vi "CRYSet Cursor in Default Position.vi"(8 "Intensity Graph Ref":refnum<vi>, 9 "Wave Graph Ref":refnum<vi>, 10 "XY Graph Ref":refnum<vi>, 11 "Graph Type":string) -> ()   [LabVIEW 2013]
uses:
  <vilib>/Utility/miscctls.llb/LVPointDoubleTypeDef.ctl
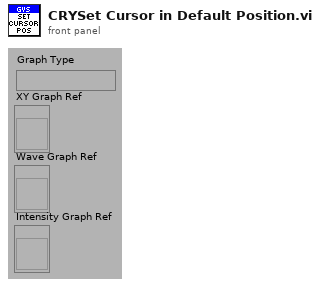
[diagram p1: front panel]
types:
  T1 = typedef "LVPointDoubleTypeDef.ctl" = cluster{"X":dbl, "Y":dbl}
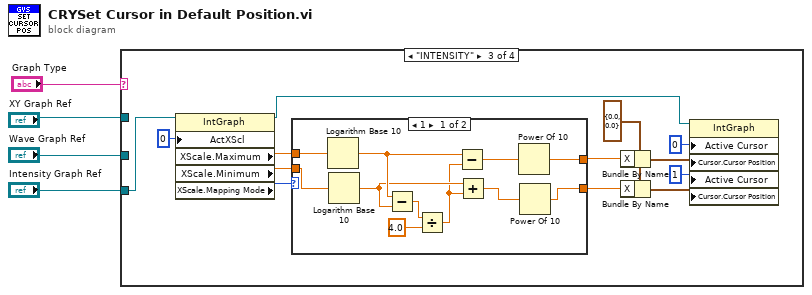
[diagram p0: block diagram]
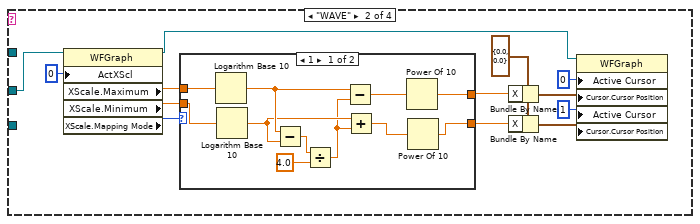
[diagram p3: hidden frame]
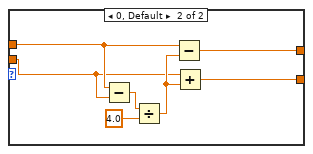
[diagram p4: hidden frame]
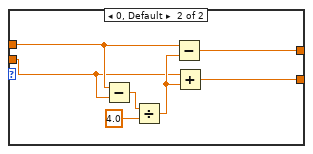
[diagram p5: hidden frame]
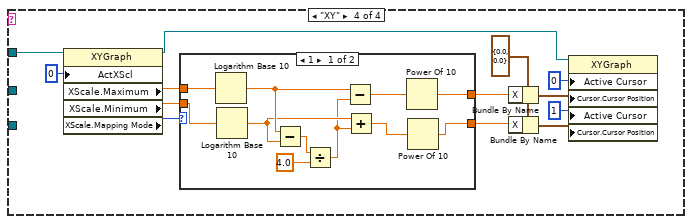
[diagram p6: hidden frame]
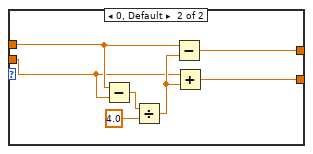
[diagram p7: hidden frame]
diagram:
  n1 = case shown="\"INTENSITY\"" "Graph Type" {
    tunnel: "XY Graph Ref" -> [_ _ _ w67]
    tunnel: "Intensity Graph Ref" -> [_ _ w36 _]
    tunnel: "Wave Graph Ref" -> [_ w5 _ _]
    frame Default {
    }
    frame "WAVE" {
      w12 = T1 {"X"=0.0, "Y"=0.0} ("Cursor.Cursor Position")
      n2 = property on="Property Node" class="WFGraph"(reference=w5, "ActXScl"=0 ("Active X Scale")) -> (reference out=w10:refnum<vi>, "XScale.Maximum"=w17:dbl, "XScale.Minimum"=w16:dbl, "XScale.Mapping Mode"=w9:u8)  [unwired: 1 in, 1 out]
      n3 = case shown="1" w9 {
        tunnel: w17 -> [w27 w32]
        tunnel: w16 -> [w25 w31]
        tunnel: [w19 w29] -> w13
        tunnel: [w18 w30] -> w11
        frame 1 {
          n4 = Logarithm Base 10(1:w27) -> (0:w28:dbl)
          n5 = Logarithm Base 10(1:w25) -> (0:w26:dbl)
          n6 = Subtract(x=w28, y=w26) -> (x-y=w22:dbl)
          n7 = Divide(x=w22, y=4.0) -> (x/y=w24:dbl)
          n8 = Subtract(x=w28, y=w24) -> (x-y=w21:dbl)
          n9 = Add(x=w26, y=w24) -> (x+y=w20:dbl)
          n10 = Power Of 10(x=w21) -> (10^x=w19:dbl)
          n11 = Power Of 10(x=w20) -> (10^x=w18:dbl)
        }
        frame 0, Default {
          n12 = Subtract(x=w32, y=w31) -> (x-y=w33:dbl)
          n13 = Divide(x=w33, y=4.0) -> (x/y=w35:dbl)
          n14 = Subtract(x=w32, y=w35) -> (x-y=w29:dbl)
          n15 = Add(x=w31, y=w35) -> (x+y=w30:dbl)
        }
      }
      n16 = Bundle By Name(cluster=w12, "X"=w13) -> (w8:T1)
      n17 = Bundle By Name(cluster=w12, "X"=w11) -> (w6:T1)
      n18 = property on="Property Node" class="WFGraph"(reference=w10, "Active Cursor"=u32 0, "Cursor.Cursor Position"=w8, "Active Cursor"=u32 1, "Cursor.Cursor Position"=w6) -> ()  [unwired: 1 in, 2 out]
    }
    frame "INTENSITY" {
      w43 = T1 {"X"=0.0, "Y"=0.0} ("Cursor.Cursor Position")
      n19 = property on="Property Node" class="IntGraph"(reference=w36, "ActXScl"=0 ("Active X Scale")) -> (reference out=w41:refnum<vi>, "XScale.Maximum"=w48:dbl, "XScale.Minimum"=w47:dbl, "XScale.Mapping Mode"=w40:u8)  [unwired: 1 in, 1 out]
      n20 = case shown="1" w40 {
        tunnel: w48 -> [w58 w63]
        tunnel: w47 -> [w56 w62]
        tunnel: [w50 w60] -> w44
        tunnel: [w49 w61] -> w42
        frame 1 {
          n21 = Logarithm Base 10(1:w58) -> (0:w59:dbl)
          n22 = Logarithm Base 10(1:w56) -> (0:w57:dbl)
          n23 = Subtract(x=w59, y=w57) -> (x-y=w53:dbl)
          n24 = Divide(x=w53, y=4.0) -> (x/y=w55:dbl)
          n25 = Subtract(x=w59, y=w55) -> (x-y=w52:dbl)
          n26 = Add(x=w57, y=w55) -> (x+y=w51:dbl)
          n27 = Power Of 10(x=w52) -> (10^x=w50:dbl)
          n28 = Power Of 10(x=w51) -> (10^x=w49:dbl)
        }
        frame 0, Default {
          n29 = Subtract(x=w63, y=w62) -> (x-y=w64:dbl)
          n30 = Divide(x=w64, y=4.0) -> (x/y=w66:dbl)
          n31 = Subtract(x=w63, y=w66) -> (x-y=w60:dbl)
          n32 = Add(x=w62, y=w66) -> (x+y=w61:dbl)
        }
      }
      n33 = Bundle By Name(cluster=w43, "X"=w44) -> (w39:T1)
      n34 = Bundle By Name(cluster=w43, "X"=w42) -> (w37:T1)
      n35 = property on="Property Node" class="IntGraph"(reference=w41, "Active Cursor"=u32 0, "Cursor.Cursor Position"=w39, "Active Cursor"=u32 1, "Cursor.Cursor Position"=w37) -> ()  [unwired: 1 in, 2 out]
    }
    frame "XY" {
      w75 = T1 {"X"=0.0, "Y"=0.0} ("Cursor.Cursor Position")
      n36 = property on="Property Node" class="XYGraph"(reference=w67, "ActXScl"=0 ("Active X Scale")) -> (reference out=w70:refnum<vi>, "XScale.Maximum"=w79:dbl, "XScale.Minimum"=w78:dbl, "XScale.Mapping Mode"=w73:u8)  [unwired: 1 in, 1 out]
      n37 = case shown="1" w73 {
        tunnel: w79 -> [w89 w94]
        tunnel: w78 -> [w87 w93]
        tunnel: [w81 w91] -> w76
        tunnel: [w80 w92] -> w74
        frame 1 {
          n38 = Logarithm Base 10(1:w89) -> (0:w90:dbl)
          n39 = Logarithm Base 10(1:w87) -> (0:w88:dbl)
          n40 = Subtract(x=w90, y=w88) -> (x-y=w84:dbl)
          n41 = Divide(x=w84, y=4.0) -> (x/y=w86:dbl)
          n42 = Subtract(x=w90, y=w86) -> (x-y=w83:dbl)
          n43 = Add(x=w88, y=w86) -> (x+y=w82:dbl)
          n44 = Power Of 10(x=w83) -> (10^x=w81:dbl)
          n45 = Power Of 10(x=w82) -> (10^x=w80:dbl)
        }
        frame 0, Default {
          n46 = Subtract(x=w94, y=w93) -> (x-y=w95:dbl)
          n47 = Divide(x=w95, y=4.0) -> (x/y=w97:dbl)
          n48 = Subtract(x=w94, y=w97) -> (x-y=w91:dbl)
          n49 = Add(x=w93, y=w97) -> (x+y=w92:dbl)
        }
      }
      n50 = Bundle By Name(cluster=w75, "X"=w76) -> (w69:T1)
      n51 = Bundle By Name(cluster=w75, "X"=w74) -> (w68:T1)
      n52 = property on="Property Node" class="XYGraph"(reference=w70, "Active Cursor"=u32 0, "Cursor.Cursor Position"=w69, "Active Cursor"=u32 1, "Cursor.Cursor Position"=w68) -> ()  [unwired: 1 in, 2 out]
    }
  }
